vi "SetBounds.vi"(0 "upper_bound":dbl format="%#_13g", 1 "lower_bound":dbl format="%#_13g", 4 "LabVIEW Web Service Request":refnum<class "Web Request.lvclass">) -> ()   [LabVIEW 2016]
uses:
  <vilib>/wsapi/Web Request.lvclass
  <vilib>/wsapi/NI_WebServices.lvlib
panel:
  out "Intensity Graph":dbl[][](graph)
  # "Use the Web Service Request input terminal to call the VIs on the Web Services palette. Do not remove it from the connector pane unless you don't need access to the palette."
  # "Each additional control wired to the connector pane will be available as an input in the URL. To include an indicator in terminal-mode output (the default setting), it must also be wired to the connector pane."
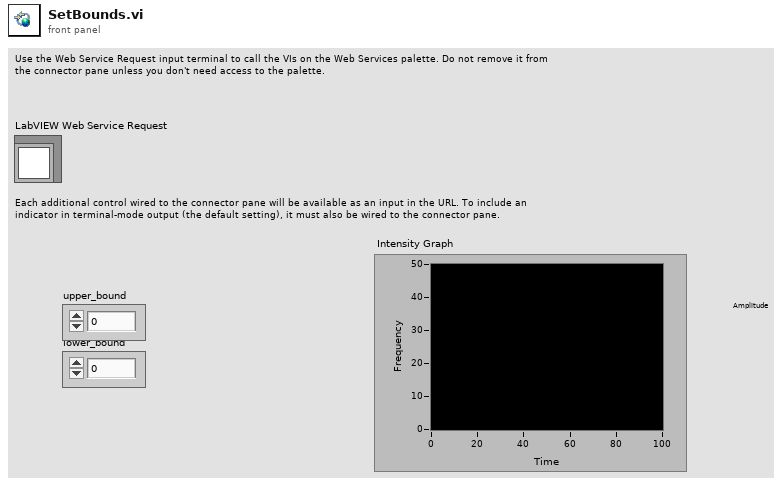
[diagram p1: front panel]
types:
  T1 = typedef "imagedata.ctl" = cluster{"image type":i32, "image depth":i32, "image":u8[], "mask":u8[], "colors":u32[], "Rectangle":cluster{"left":i16, "top":i16, "right":i16, "bottom":i16}}
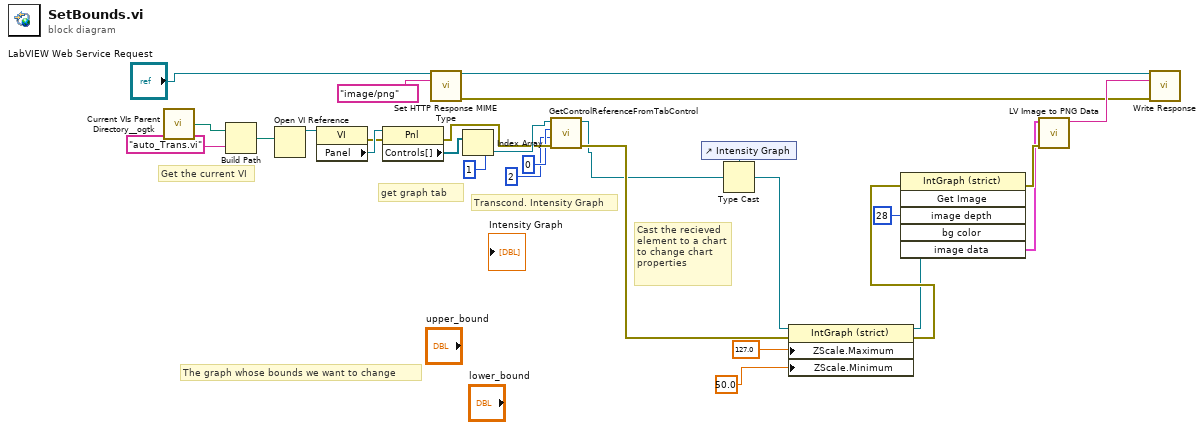
[diagram p0: block diagram]
diagram:
  # "Cast the recieved element to a chart to change chart properties"
  # "Transcond. Intensity Graph"
  # "Get the current VI"
  # "get graph tab"
  # "The graph whose bounds we want to change"
  n1 = call <userlib>:"Current VIs Parent Directory__ogtk.vi"() -> ("Parent Directory (+ Relative)"=w23:path)  [unwired: 5 in]
  n2 = Build Path(base path=w23, name or relative path="auto_Trans.vi") -> (appended path=w21:path)
  n3 = Open VI Reference(vi path=w21) -> (vi reference=w24:refnum<vi>)  [unwired: 5 in, 1 out]
  n4 = property class="VI"(reference=w24) -> (error out=w11:errorcluster, "Panel"=w20:refnum<vi>)  [unwired: 1 in, 1 out]
  n5 = property class="Pnl"(reference=w20, error in=w11) -> (error out=w12:errorcluster, "Controls[]"=w19:refnum<vi>[])  [unwired: 1 out]
  n6 = call <vilib>:"Set HTTP Response MIME Type.vi"("LabVIEW Web Service Request"="LabVIEW Web Service Request", "MIME type (text/html)"="image/png") -> ("LabVIEW Web Service Request out"=w27:refnum<class "Web Request.lvclass">, "error out"=w25:errorcluster)  [unwired: 12 in]
  n7 = Index Array(array=w19, index=1) -> (element=w14:refnum<vi>)
  n8 = call "GetControlReferenceFromTabControl.vi"("error in (no error)"=w12, "control"=2 ("page"), "page"=0 ("control"), "Ctl Refnum"=w14) -> ("error out"=w13:errorcluster, "element"=w2:refnum<vi>)  [unwired: 6 in]
  n9 = control-ref of="Intensity Graph"() -> (w16:refnum<vi>)
  n10 = Type Cast(type=w16, x=w2) -> (*(type *) &x=w15:refnum<vi>)
  n11 = property class="IntGraph (strict)"(reference=w15, error in=w13, "ZScale.Maximum"=127.0 ("upper_bound"), "ZScale.Minimum"=50.0 ("upper_bound")) -> (reference out=w1:refnum<vi>, error out=w8:errorcluster)
  n12 = invoke class="IntGraph (strict)" method="Get Image"(reference=w1, error in=w8, "image depth"=28 ("Image Depth")) -> (error out=w7:errorcluster, "image data"=w6:T1)  [unwired: 3 in, 4 out]
  n13 = call <vilib>:"LV Image to PNG Data.vi"("error in (no error)"=w7, "image data"=w6) -> ("png data"=w26:string)  [unwired: 8 in, 1 out]
  n14 = call <vilib>:"Write Response.vi"("LabVIEW Web Service Request"=w27, "response string"=w26, "error in (no error)"=w25) -> ()  [unwired: 11 in, 2 out]
